vi "MDAQ_SaveCVSpectrums.vi"(5 "User Comment":string, 7 "Sample Name":string, 8 "error in":errorcluster, 9 "Control Cluster":T1 {"CV"."Temperature Array" scale=0.0..100.0}, 10 "Status_Cluster":T3 {"GATESTOP" format="%04x"; "GATESTRT" format="%04x"; "AMPLITUDE" format="%04x"; "M_CYCLES" format="%04x"; "N_CYCLES" format="%04x"; "STEP" format="%04x"; "BASE" format="%04x"; "CHAN" format="%04x"}, 11 "file path (use dialog)":path) -> (0 "error out":errorcluster, 1 "Control Cluster Out":T1 {"CV"."Temperature Array" scale=0.0..100.0}, 2 "Status_Cluster Out":T3 {"GATESTOP" format="%04x"; "GATESTRT" format="%04x"; "AMPLITUDE" format="%04x"; "M_CYCLES" format="%04x"; "N_CYCLES" format="%04x"; "STEP" format="%04x"; "BASE" format="%04x"; "CHAN" format="%04x"})   [LabVIEW 2021]
uses:
  GUI_Def.ctl
  Mode_Enum.ctl
  Status_Cluster.ctl
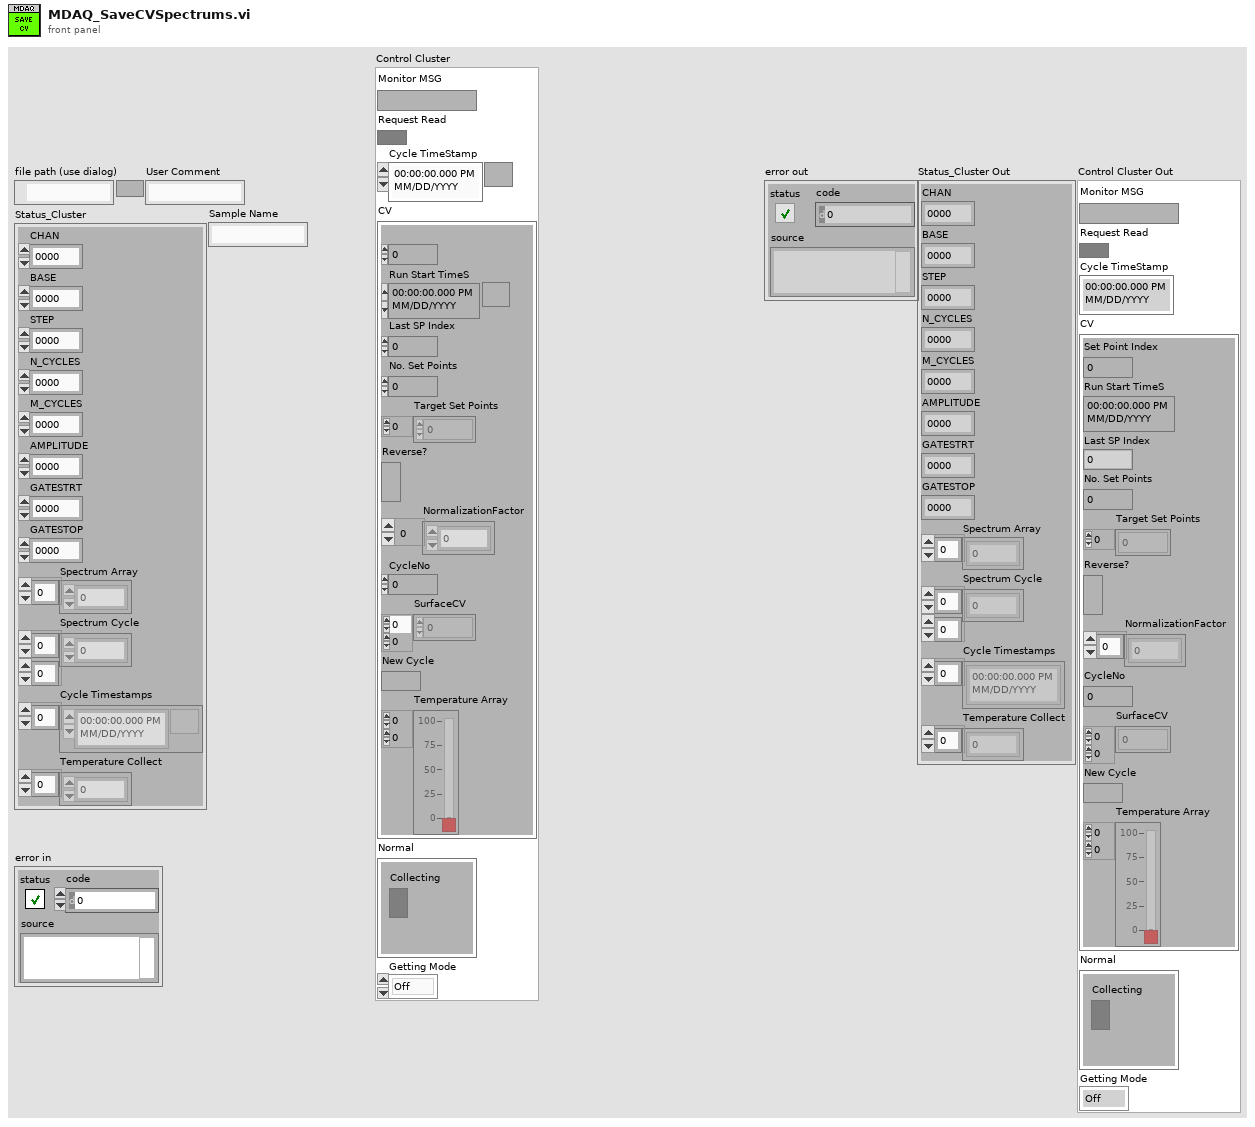
[diagram p1: front panel]
types:
  T1 = typedef "GUI_Def.ctl" = cluster{"Monitor MSG":string, "Request Read":bool, "Cycle TimeStamp":timestamp, "CV":cluster{"Set Point Index":u32, "Run Start TimeS":timestamp, "Last SP Index":u32, "No. Set Points":u32, "Target Set Points":i32[], "Reverse?":bool, "NormalizationFactor":i32[], "CycleNo":i32, "SurfaceCV":dbl[][], "New Cycle":bool, "Temperature Array":dbl[][]}, "Normal":cluster{"Collecting":bool}, "Getting Mode":T2}
  T2 = typedef "Mode_Enum.ctl" = enum16{"Off", "Normal", "CV+Temp", "CV"}
  T3 = typedef "Status_Cluster.ctl" = cluster{"CHAN":u32, "BASE":u32, "STEP":u32, "N_CYCLES":u32, "M_CYCLES":u32, "AMPLITUDE":u32, "GATESTRT":u32, "GATESTOP":u32, "Spectrum Array":u32[], "Spectrum Cycle":u32[][], "Cycle Timestamps":timestamp[], "Temperature Collect":dbl[]}
  T4 = enum16{"open", "replace", "create", "open or create", "replace or create", "replace or create with confirmation"}
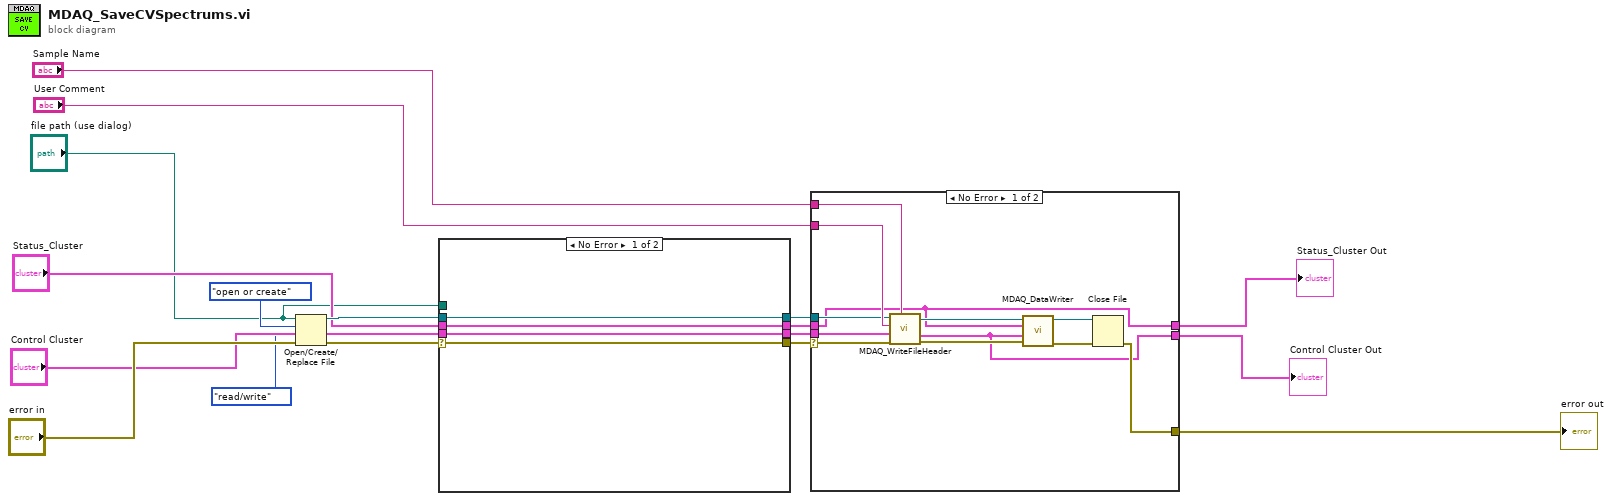
[diagram p0: block diagram]
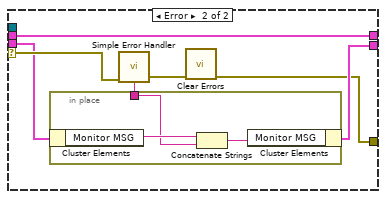
[diagram p2: hidden frame]
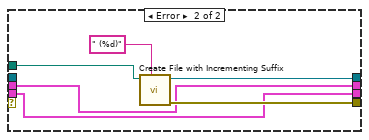
[diagram p3: hidden frame]
diagram:
  n1 = Open/Create/Replace File(file path (use dialog)="file path (use dialog)", error in="error in", operation (0:open)=T4."open or create", access (0:read/write)=enum16{"read/write", "read-only", "write-only"}."read/write") -> (refnum out=w14:refnum<file>, error out=w15:errorcluster)  [unwired: 2 in, 1 out]
  n2 = case shown="No Error" w15 {
    selector: w15 -> [w21 _]
    tunnel: w14 -> [w20 _]
    tunnel: [w21 w24] -> w13
    tunnel: [w20 w25] -> w12
    tunnel: "Control Cluster" -> [w19 w22]
    tunnel: [w19 w22] -> w8
    tunnel: "Status_Cluster" -> [w18 w23]
    tunnel: [w18 w23] -> w6
    tunnel: "file path (use dialog)" -> [_ w27]
    frame No Error {
    }
    frame Error {
      n3 = call <vilib>:"Create File with Incrementing Suffix.vi"("format string (\" (%d)\")"=" (%d)" ("format string (\" (%d)\")"), "file path"=w27) -> ("error out"=w24:errorcluster, "refnum out"=w25:refnum<file>)  [unwired: 7 in, 1 out]
    }
  }
  n4 = case shown="No Error" w13 {
    selector: w13 -> [w36 w46]
    tunnel: w12 -> [w37 _]
    tunnel: "Sample Name" -> [w39 _]
    tunnel: "User Comment" -> [w38 _]
    tunnel: w8 -> [w35 w44]
    tunnel: w6 -> [w29 w45]
    tunnel: [w29 w45] -> w3
    tunnel: [w28 w42] -> w2
    tunnel: [w32 w40] -> w4
    frame No Error {
      n5 = call "MDAQ_WriteFileHeader.vi"("Sample Name"=w39, "error in"=w36, "Control Cluster"=w35, "User Comment"=w38, "FileRef In"=w37) -> ("error out"=w33:errorcluster, "Control Cluster Out"=w28:T1, "refnum out"=w34:refnum<file>)  [unwired: 4 in]
      n6 = call "MDAQ_DataWriter.vi"("error in"=w33, "Control Cluster"=w28, "Status_Cluster"=w29, "FileRef In"=w34) -> ("error out"=w30:errorcluster, "refnum out"=w31:refnum<file>)  [unwired: 6 in]
      n7 = Close File(refnum=w31, error in=w30) -> (error out=w32:errorcluster)  [unwired: 1 out]
    }
    frame Error {
      n8 = call <vilib>:"Simple Error Handler.vi"("error in (no error)"=w46) -> ("error out"=w41:errorcluster, "message"=w43:string)  [unwired: 4 in, 3 out]
      n9 = in-place {
        in-place-border: w43 -> [w48]
        n10 = in-place-cluster #1(w44) -> ("Monitor MSG"=w49:string)
        n11 = Concatenate Strings(w49, w48) -> (w47:string)
        n12 = in-place-cluster #1("Monitor MSG"=w47) -> (w42:T1)
      }
      n13 = call <vilib>:"Clear Errors.vi"("error in (no error)"=w41) -> ("error out"=w40:errorcluster)  [unwired: 5 in, 1 out]
    }
  }
  "error out" <- w4
  "Status_Cluster Out" <- w3
  "Control Cluster Out" <- w2
